vi "play-AFM-CS-imaging_v2.vi"() -> ()   [LabVIEW 2017]
uses:
  z-axis-params.ctl
  controls/boolean_info.ctl
  <userlib>/_matio/level5/Public/MAT-File Data Types.ctl
  <vilib>/userdefined/High Color/nirio_resource_hc.ctl
  controls/expMetaData.ctl
  <vilib>/Utility/file.llb/Read Delimited Spreadsheet (DBL).vi
  <vilib>/FPGAPlugInAG/cRIO-9082/niLvFpga_Open_cRIO-9082.vi
  <vilib>/rvi/interface/common/dynamic/niFpgaDynamicAddResources.vi
  <vilib>/FPGAPlugInAG/Dynamic/niLvFpga_Reset_Dynamic.vi
  <vilib>/rvi/interface/common/niFpgaWaitOnOcc.vi
  <vilib>/Utility/error.llb/Error Cluster From Error Code.vi
  <vilib>/rvi/errors/niLvFpgaAdjustHostInterfaceError.vi
  <vilib>/FPGAPlugInAG/Dynamic/niLvFpga_Run_Dynamic.vi
  <vilib>/Utility/file.llb/Write Delimited Spreadsheet (DBL).vi
  <vilib>/FPGAPlugInAG/Dynamic/niLvFpga_Close_Dynamic.vi
  <userlib>/_matio/level5/Public/Write/Append Data Element.llb/Append Data Element (Anything).vi
  <vilib>/rvi/interface/nirviOpenFPGA/nirviOpenFPGA.xnode
  FPGA Bitfiles/afmimagingcontro_FPGATargetSPARTA_cs-scanningv2.lvbitx
  <vilib>/rvi/interface/nirviMethod/nirviMethod.xnode
  <vilib>/rvi/interface/nirviReadWriteControl/nirviReadWriteControl.xnode
  <vilib>/rvi/interface/nirviCloseFPGA/nirviCloseFPGA.xnode
  <vilib>/FPGAPlugInAG/Dynamic/niLvFpga_ConfigureFifo_Dynamic.vi
  <vilib>/rvi/errors/niLvFpgaMergeErrorWithErrorCode.vi
  <vilib>/rvi/interface/Simulation/niFpgaSimulationCallBeginRW.vi
  <vilib>/FPGAPlugInAG/Dynamic/niLvFpga_ReadFifo_Dynamic.vi
  NiFpgaLv.dll
  <userlib>/_matio/level5.lvlib
  <vilib>/FPGAPlugInAG/Dynamic/niLvFpga_WriteFifo_Dynamic.vi
panel:
  out "xy_ref":fxp<+/-,16,5>[](array[numeric])
  out "xy_k":fxp<+/-,16,5>[](array[numeric])
  out "input-data-path":path
  in  "Kiz_down":sgl=0.001
  in  "max_Z_settle_samples":i16=5000
  out "boolean \nindicators":T1
  out "CS Time":dbl
  out "Current Case":i16
  out "state times":dbl[](array[numeric])
  out "iter":i32
  out "entity-index":i16
  out "x = 0?":bool
  out "Numeric":i32
  out "error out 2":errorcluster
  in  "Tab Control":T2(tab)
  in  "init Z up":sgl step=0.5
  in  "trigger-0":bool
  in  "numEntities":i16
  in  "data-root":path=path "C:/Users/arnold/Documents/labview/afm_imaging/data/cs-data/20microns/parents"
  in  "z-axis-params":T3={"TOL"=0.3, "ramp_rate"=-5e-05, "z_u_max"=5.0, "setpoint"=0.0, "Ki"=0.01, "Z_error_threshold"=0.05, "Z_settled_samples_threshold "=500, "z_UP"=1.5, "zup_N"=500, "TF Order"=1, "Num"=[1.0, 0.0, 0.0, 0.0, 0.0, 0.0, 0.0, 0.0, 0.0], "Den"=[1.0, 0.0, 0.0, 0.0, 0.0, 0.0, 0.0, 0.0, 0.0]} {"Z_error_threshold" format="%#_13g"; "ramp_rate" format="%#_4g"; "TOL" format="%#_13g"}
  in  "step_down_frac":fxp<+,8,1>=1.0
  in  "input-file-name":string="cs-traj-z-bounce.csv"
  out "output-data-path":path
  out "output-meta-data-path":path
  in  "note-blob":string
  in  "overwrite":bool
  in  "TsTicks":u32=1600
  in  "Ki-xy":sgl=0.005
  in  "collect all":bool=TRUE
  in  "collect move":bool
  in  "xy settled-samples\n threshold":i16=200
  in  "xy error-threshold":sgl=0.1
  out "number-settled-samples-x":i16
  out "number-settled-samples-y":i16
  out "case-selected":i16
  out "number-settled-samples-Z":i16
  out "size(s)":i32
  out "nsamps":i32
  out "elements left":i32=1
  out "y iter":i32
  out "size(s) 2":i32[](array[numeric])
  out "Array":i32[][](array[numeric])
  out "z-control":dbl[](graph)
  out "x-axis":dbl[](graph)
  out "z-error":dbl[](graph)
  out "y-axis":dbl[](graph)
  in  "STOP":bool
  # "- If collect all = fasle and collect move = false,\nwe only collect measurement data.\n- If collect all = false, and collect move = true,\nwe collect measurement and move data.\n- If collect all = true, we collect everything."
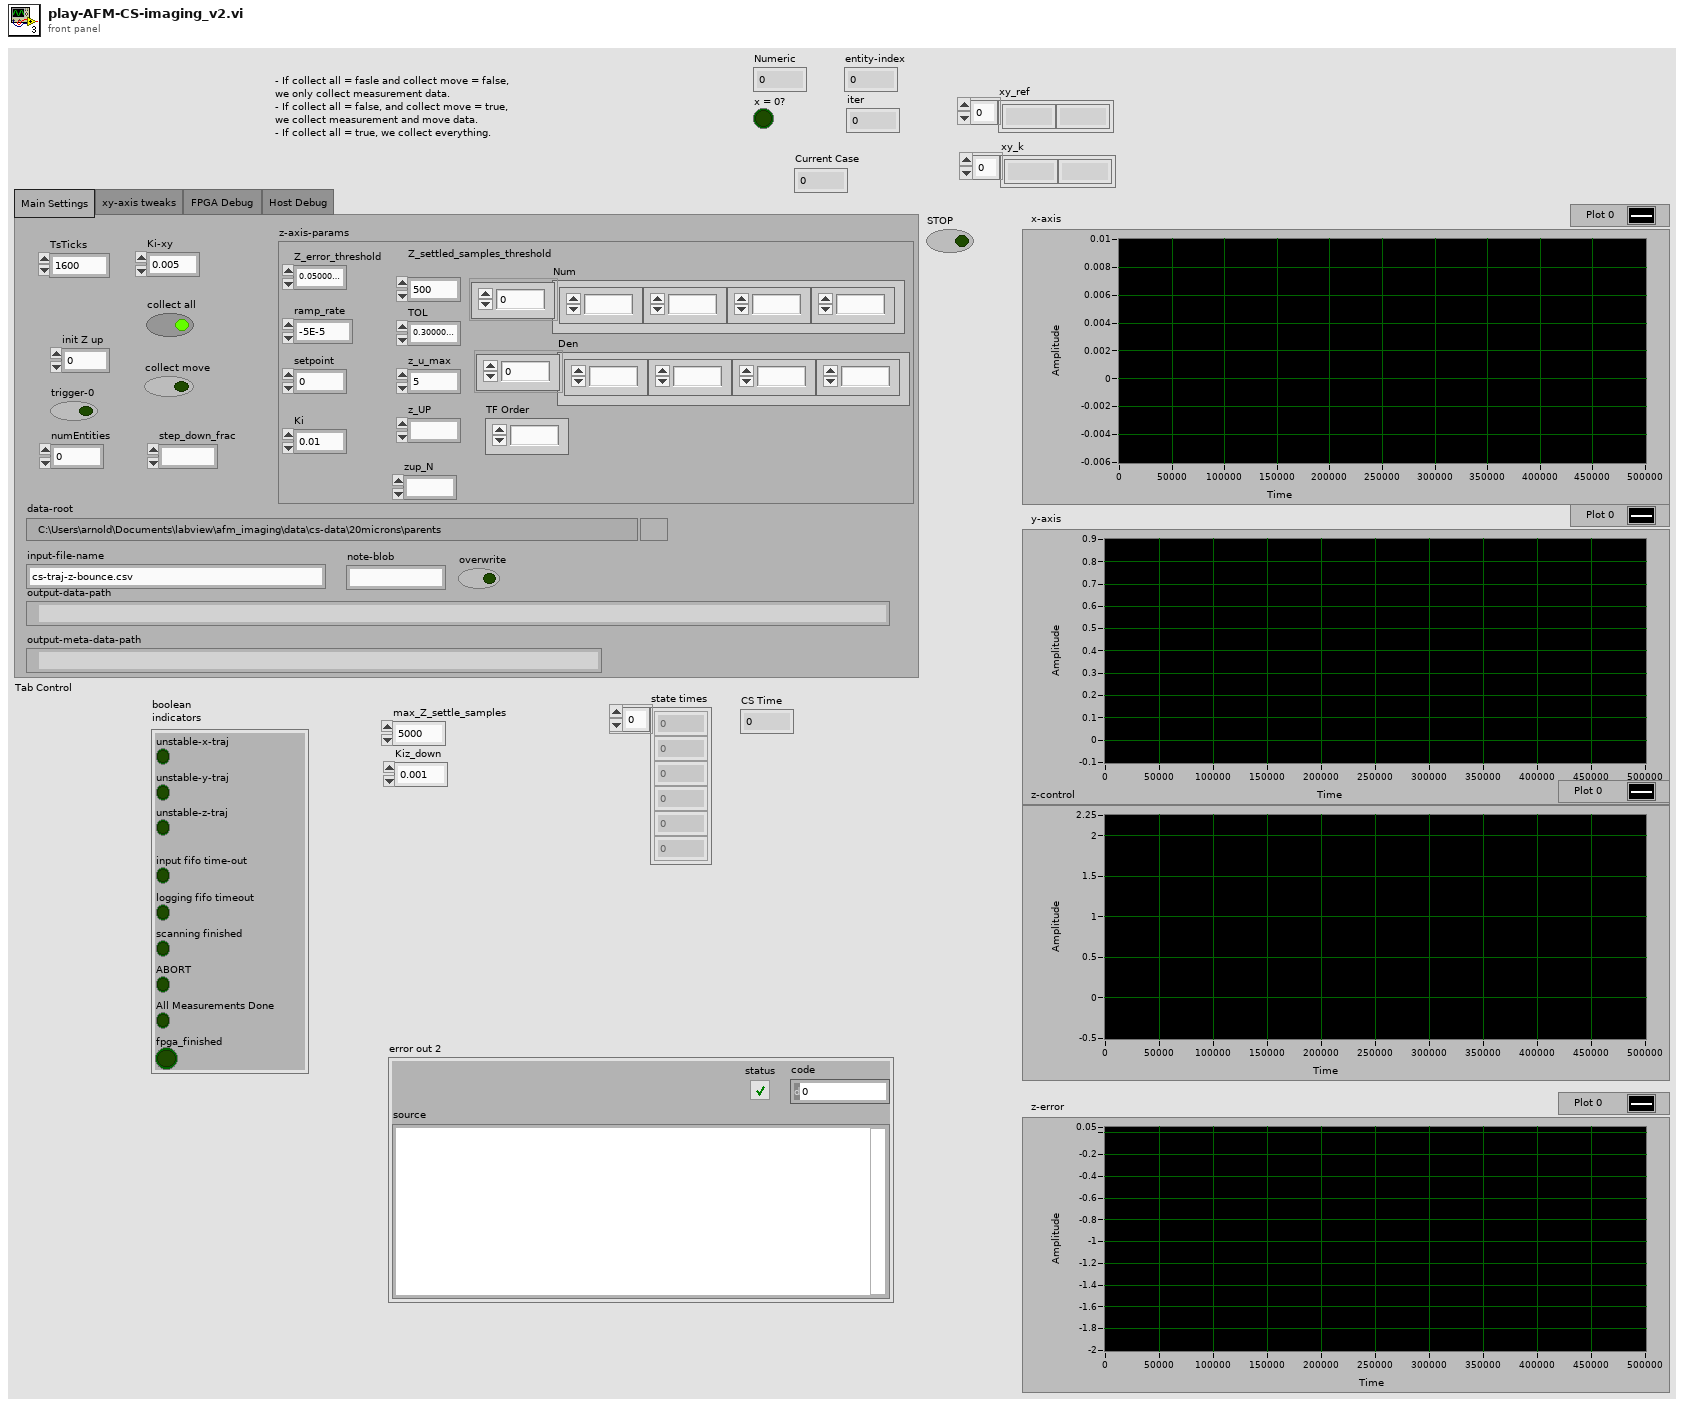
[diagram p1: front panel]
types:
  T1 = typedef "boolean_info.ctl" = cluster{"unstable-z-traj":bool, "input fifo time-out":bool, "logging fifo timeout":bool, "scanning finished":bool, "unstable-x-traj":bool, "unstable-y-traj":bool, "ABORT":bool, "All Measurements Done":bool, "fpga_finished":bool}
  T2 = enum32{"Main Settings", "xy-axis tweaks", "FPGA Debug ", "Host Debug"}
  T3 = typedef "z-axis-params.ctl" = cluster{"TOL":sgl, "ramp_rate":sgl, "z_u_max":sgl, "setpoint":sgl, "Ki":sgl, "Z_error_threshold":sgl, "Z_settled_samples_threshold ":i16, "z_UP":fxp<+/-,16,5>, "zup_N":i16, "TF Order":i32, "Num":sgl[], "Den":sgl[]}
  T4 = typedef "level5.lvlib/MAT-File Data Types.ctl" = enum32{"_invalid", "miINT8", "miUINT8", "miINT16", "miUINT16", "miINT32", "miUINT32", "miSINGLE", "_reserved_1", "miDOUBLE", "_reserved_2", "_reserved_3", "miINT64", "miUINT64", "miMATRIX", "miCOMPRESSED", "miUTF8", "miUTF16", "miUTF32"}
  T5 = typedef "nirio_resource_hc.ctl" = tag
  T6 = cluster{"unstable-z-traj":bool, "input fifo time-out":bool, "logging fifo timeout":bool, "scanning finished":bool, "unstable-x-traj":bool, "unstable-y-traj":bool, "ABORT":bool, "All Measurements Done":bool, "fpga_finished":bool}
  T7 = enum16{"open", "replace", "create", "open or create", "replace or create", "replace or create with confirmation"}
  T8 = typedef "expMetaData.ctl" = cluster{"xy_error_threshold":sgl, "xy_settled_samples_threshold":i16, "Ki_xy":sgl, "state_counts":dbl[], "TOL":sgl, "ramp_rate":sgl, "z_u_max":sgl, "setpoint":sgl, "Ki":sgl, "Z_error_threshold":sgl, "Z_settled_samples_threshold ":i16, "z_UP":sgl, "zup_N":i16, "Num":sgl[], "Den":sgl[], "max_Z_settle_samples":i16, "Kiz_down":sgl, "do_xy_CL":bool, "do_Alt_Ztrigger":bool, "output-data-path":path, "input-data-path":path}
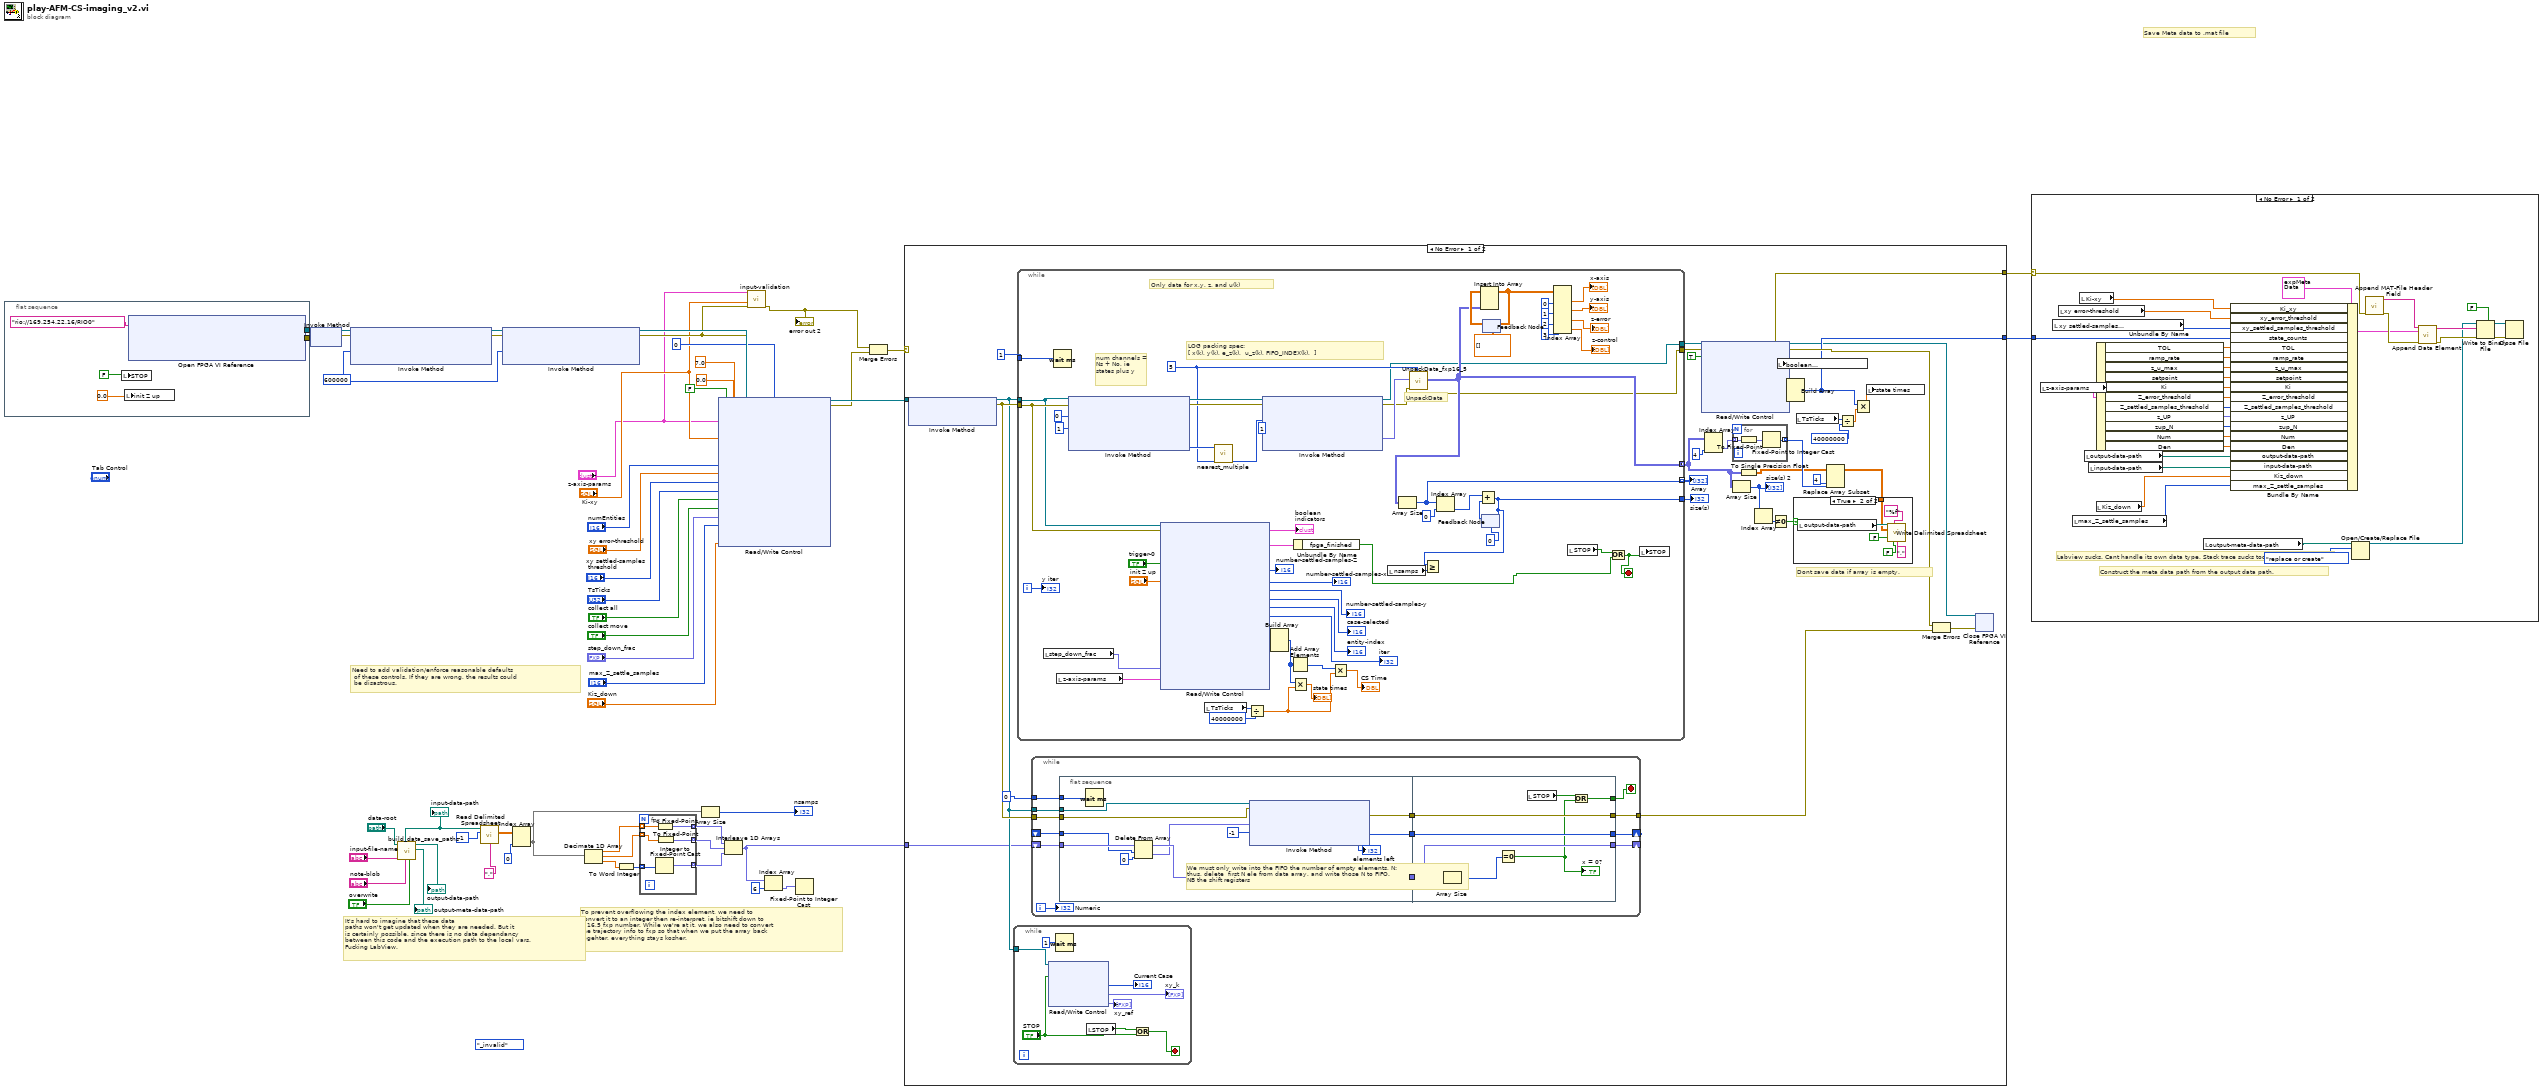
[diagram p0: block diagram]
diagram:
  (unwired) MAT-File_Data_Types."_invalid" ("MAT-File Data Types")
  w52 = 600000
  # "It's hard to imagine that these data\npaths won't get updated when they are needed. But it \nis certainly possible, since there is no data dependancy \nbetween this code and the execution path to the local vars.\nFucking LabView."
  # "Save Meta data to .mat file"
  # "To prevent overflowing the index element, we need to \nconvert it to an integer then re-interpret, ie bitshift down to \na 16,5 fxp number. While we're at it, we also need to convert\nthe trajectory info to fxp so that when we put the array back\ntogehter, everything stays kosher."
  # "Need to add validation/enforce reasonable defaults\n of these controls. If they are wrong, the results could\n be disastrous."
  n1 = flat-sequence {
    tunnel: [w58] -> w51
    tunnel: [w57] -> w50
    frame #0 {
      n2 = local write "STOP"(FALSE) -> ()
      n3 = local write "init Z up"(0.0) -> ()
      n4 = xnode "Open FPGA VI Reference"("resource name"=T5 "rio://169.254.22.16/RIO0") -> ("FPGA VI Reference Out"=w58:refnum<k20>, "error out"=w57:errorcluster)  [unwired: 1 in]
    }
  }
  n5 = xnode "Invoke Method"("FPGA VI Reference In"=w51, "error in"=w50) -> ("FPGA VI Reference Out"=w45:refnum<k20>, "error out"=w44:errorcluster)
  n6 = xnode "Invoke Method"("FPGA VI Reference In"=w45, "error in"=w44, "Requested Depth"=w52) -> ("FPGA VI Reference Out"=w47:refnum<k20>, "error out"=w48:errorcluster)  [unwired: 1 out]
  n7 = call "build_data_save_paths.vi"("overwrite"="overwrite", "note-blob"="note-blob", "base-file-name"="input-file-name", "data-root"="data-root") -> ("output-meta-data-path"=→"output-meta-data-path":path, "output-data-path"=→"output-data-path":path, "input-data-path"=w6:path)  [unwired: 3 in, 2 out]
  "input-data-path" <- w6
  n8 = call-poly <vilib>:"Read Delimited Spreadsheet.vi"("file path (dialog if empty)"=w6, "number of rows (all:-1)"=-1, "delimiter (\\t)"=",") -> ("all rows"=w39:dbl[][])  [unwired: 7 in, 5 out]
  n9 = xnode "Invoke Method"("FPGA VI Reference In"=w47, "error in"=w48, "Requested Depth"=w52) -> ("FPGA VI Reference Out"=w53:refnum<k20>, "error out"=w31:errorcluster)  [unwired: 1 out]
  n10 = Index Array(array=w39, index (col)=0 ("dimension size")) -> (element=w17:dbl[])  [unwired: 1 in]
  n11 = Decimate 1D Array(w17) -> (w25:dbl[], w24:dbl[], w26:dbl[])
  n12 = To Word Integer(number=w26) -> (16bit integer=w23:i16[])
  n13 = for {
    tunnel: w25 -> [w64] mode=indexing
    tunnel: w24 -> [w63] mode=indexing
    tunnel: [w62] -> w21 mode=indexing
    tunnel: [w61] -> w22 mode=indexing
    tunnel: w23 -> [w60] mode=indexing
    tunnel: [w59] -> w20 mode=indexing
    n14 = Integer to Fixed-Point Cast(integer=w60) -> (fixed-point=w59:fxp<+/-,16,5>)  [unwired: 1 in]
    n15 = To Fixed-Point(number=w64) -> (fixed-point=w61:fxp<+/-,16,5>)  [unwired: 1 in]
    n16 = To Fixed-Point(number=w63) -> (fixed-point=w62:fxp<+/-,16,5>)  [unwired: 1 in]
  }
  n17 = Array Size(array=w17) -> (size(s)=→"nsamps":i32)
  n18 = xnode "Read/Write Control"("FPGA VI Reference In"=w53, "error in"=w31, "initial case"=i16 0, "z-axis-params"="z-axis-params", "xy-bound"=sgl 7.0, "Ki-xy"="Ki-xy", "init Z up"=sgl 0.0 ("u(0)"), "trigger-0"=FALSE, "numEntities"="numEntities", "xy-error-threshold"="xy error-threshold", "settled-samples threshold"="xy settled-samples\n threshold", "TsTicks"="TsTicks", "collect all"="collect all", "collect move"="collect move", "step_down_frac"="step_down_frac", "max_Z_settle_samples"="max_Z_settle_samples", "Kiz_down"="Kiz_down") -> ("FPGA VI Reference Out"=w46:refnum<k20>, "error out"=w28:errorcluster)  [unwired: 1 out]
  n19 = Interleave 1D Arrays(w22, w21, w20) -> (w16:fxp<+/-,16,5>[])
  n20 = call "input-validation.vi"("error constant"=w31, "Ki-xy"="Ki-xy", "z-axis-params"="z-axis-params") -> ("error out"=w27:errorcluster)  [unwired: 8 in]
  "error out 2" <- w27
  n21 = Index Array(array=w16, index=6) -> (element=w19:fxp<+/-,16,5>)
  n22 = Fixed-Point to Integer Cast(1:w19) -> ()  [unwired: 1 out]
  n23 = Merge Errors(w27, w28) -> (w1:errorcluster)
  n24 = case shown="No Error" w1 {
    selector: w1 -> [_ w209]
    tunnel: w46 -> [w99 _]
    tunnel: w16 -> [w97 _]
    tunnel: [w96 w209] -> w13
    tunnel: [w95 _] -> w12
    frame No Error {
      # "Dont save data if array is empty."
      n25 = xnode "Invoke Method"("FPGA VI Reference In"=w99) -> ("FPGA VI Reference Out"=w98:refnum<k20>, "error out"=w100:errorcluster)  [unwired: 2 in]
      n26 = while {
        tunnel: w98 -> [w117]
        stop <- w113 stop-if-true
        n27 = xnode "Read/Write Control"("FPGA VI Reference In"=w117, "ABORT"="STOP") -> ("Current Case"=→"Current Case":u8, "xy_k"=→"xy_k":fxp<+/-,16,5>[], "xy_ref"=→"xy_ref":fxp<+/-,16,5>[])  [unwired: 1 in, 2 out]
        n28 = Wait (ms)(milliseconds to wait=u32 1) -> ()  [unwired: 1 out]
        n29 = local read "STOP"() -> (w114:bool)
        n30 = Or(x=w114, y="STOP") -> (x .or. y?=w113:bool)
      }
      n31 = while {
        tunnel: 1 -> [w208]
        tunnel: w98 -> [w196]
        tunnel: w100 -> [w197]
        tunnel: [w161] -> w89
        tunnel: [w172] -> w80 mode=concatenating
        tunnel: [w194] -> w93
        tunnel: [w170] -> w88
        tunnel: [w187] -> w85 mode=indexing
        i -> [w195]
        stop <- w188 stop-if-true
        w173 = u32 5 ("y")
        # "LOG packing spec:\n[ x(k), y(k), e_z(k),  u_z(k), FIFO_INDEX(k),  ]"
        # "num channels = Ns + No, ie states plus y"
        # "Only data for x,y, z, and u(k)"
        # "UnpackData"
        n32 = local read "step_down_frac"() -> (w149:fxp<+,8,1>)
        n33 = Wait (ms)(milliseconds to wait=w208) -> ()  [unwired: 1 out]
        n34 = local read "z-axis-params"() -> (w150:T3)
        n35 = xnode "Invoke Method"("FPGA VI Reference In"=w196, "error in"=w197, "Number of Elements"=0 ("Timeout (ms)"), "Timeout (ms)"=1) -> ("FPGA VI Reference Out"=w204:refnum<k20>, "error out"=w205:errorcluster, "Elements Remaining"=w191:u32)  [unwired: 1 out]
        n36 = xnode "Read/Write Control"("FPGA VI Reference In"=w196, "error in"=w197, "trigger-0"="trigger-0", "init Z up"="init Z up", "step_down_frac"=w149, "z-axis-params"=w150) -> ("boolean  indicators"=w154:T6, "number-settled-samples-Z"=→"number-settled-samples-Z":i16, "number-settled-samples-x"=→"number-settled-samples-x":i16, "number-settled-samples-y"=→"number-settled-samples-y":i16, "Current Case"=→"case-selected":u8, "entity-index"=→"entity-index":i16, "iter"=→"iter":i32, "state1-count"=w166:u64, "state2-count"=w165:u64, "state3-count"=w164:u64, "state4-count"=w163:u64, "state5-count"=w162:u64)  [unwired: 1 in, 3 out]
        "boolean \nindicators" <- w154
        n37 = local read "TsTicks"() -> (w157:u32)
        n38 = call "nearest_multiple.vi"("numChan"=w173, "N"=w191) -> ("(int) y*floor(x/y)"=w190:u64)  [unwired: 9 in]
        n39 = Divide(x=w157, y=u32 40000000) -> (x/y=w152:dbl)
        n40 = xnode "Invoke Method"("FPGA VI Reference In"=w204, "error in"=w205, "Number of Elements"=w190, "Timeout (ms)"=1) -> ("FPGA VI Reference Out"=w161:refnum<k20>, "error out"=w170:errorcluster, "Data"=w171:fxp<+/-,16,5>[])  [unwired: 1 out]
        n41 = Build Array(w166, w165, w164, w163, w162) -> (w153:u64[])
        n42 = Add Array Elements(numeric array=w153) -> (sum=w158:u64)
        n43 = Multiply(x=w153, y=w152) -> (x*y=→"state times":dbl[])
        n44 = Unbundle By Name(w154) -> ("fpga_finished"=w169:bool)
        n45 = Multiply(x=w158, y=w152) -> (x*y=→"CS Time":dbl)
        n46 = local read "nsamps"() -> (w201:i32)
        n47 = call "UnpackData_fxp16_5.vi"("NumChannels"=w173, "error In"=w170, "1D Data In"=w171) -> ("2D Data Out"=w172:fxp<+/-,16,5>[][])  [unwired: 7 in, 1 out]
        n48 = Array Size(array=w172) -> (size(s)=w187:i32[])
        n49 = Index Array(array=w187, index=0) -> (element=w199:i32)
        n50 = feedback #1(0) -> (w200:i32)
        n51 = Add(x=w199, y=w200) -> (x+y=w194:i32)
        n52 = Greater Or Equal?(x=w194, y=w201) -> ()  [unwired: 1 out]
        n53 = feedback-in #1(w194) -> ()
        n54 = feedback #2(dbl[][] []) -> (w183:dbl[][])
        n55 = Insert Into Array(array=w183, new element=w172) -> (w174:dbl[][])  [unwired: 2 in]
        n56 = feedback-in #2(w174) -> ()
        n57 = Index Array(array=w174, index (col) #1=0 ("disabled index (col)"), index (col) #2=1 ("index (col)"), index (col) #3=2 ("index (col)"), index (col) #4=3 ("index (col)")) -> (element #1=→"x-axis":dbl[], element #2=→"y-axis":dbl[], element #3=→"z-error":dbl[], element #4=→"z-control":dbl[])  [unwired: 4 in]
        n58 = local read "STOP"() -> (w189:bool)
        n59 = Or(x=w189, y=w169) -> (x .or. y?=w188:bool)
        n60 = local write "STOP"(w188) -> ()
        "y iter" <- w195
      }
      "size(s)" <- w93
      "Array" <- w85
      n61 = while {
        tunnel: [w128] -> w90
        tunnel: 0 -> [w130]
        shift-right: [w124] -> _
        shift-left: _ -> [w127]
        shift-right: [w122] -> _
        shift-left: w97 -> [w129]
        tunnel: w98 -> [w121]
        tunnel: w100 -> [w120]
        i -> [w118]
        stop <- w119 stop-if-true
        n62 = flat-sequence {
          tunnel: w130 -> [w141]
          tunnel: w129 -> [w136]
          tunnel: w127 -> [w132]
          tunnel: [w139] -> w126
          tunnel: [w137] -> w125
          tunnel: [w138] -> w123
          tunnel: w121 -> [w134]
          tunnel: w120 -> [w133]
          tunnel: [w148] -> w124
          tunnel: [w145] -> w128
          tunnel: w126 -> [w145]
          tunnel: w125 -> [w148]
          tunnel: w123 -> [w146]
          tunnel: [w146] -> w122
          tunnel: [w142] -> w119
          frame #0 {
            # "We must only write into the FIFO the number of empty elements, N:\nthus, delete  first N ele from data array, and write those N to FIFO.\nNB the shift registers"
            n63 = Wait (ms)(milliseconds to wait=w141) -> ()  [unwired: 1 out]
            n64 = Delete From Array(array=w136, length=w132, index=0) -> (deleted portion=w135:fxp<+/-,16,5>[], array with subset deleted=w138:fxp<+/-,16,5>[])
            n65 = xnode "Invoke Method"("FPGA VI Reference In"=w134, "error in"=w133, "Data"=w135, "Timeout (ms)"=-1) -> ("error out"=w139:errorcluster, "Empty Elements Remaining"=w137:u32)  [unwired: 1 out]
            "elements left" <- w137
          }
          frame #1 {
            n66 = Array Size(array=w146) -> (size(s)=w147:i32)
            n67 = Equal To 0?(x=w147) -> (x = 0?=w144:bool)
            "x = 0?" <- w144
            n68 = local read "STOP"() -> (w143:bool)
            n69 = Or(x=w143, y=w144) -> (x .or. y?=w142:bool)
          }
        }
        "Numeric" <- w118
      }
      n70 = xnode "Read/Write Control"("FPGA VI Reference In"=w89, "error in"=w88, "ABORT"=TRUE) -> ("FPGA VI Reference Out"=w86:refnum<k20>, "error out"=w96:errorcluster, "boolean  indicators"=w69:T6, "state1-count"=w78:u64, "state2-count"=w77:u64, "state3-count"=w76:u64, "state4-count"=w75:u64, "state5-count"=w74:u64)
      n71 = Index Array(array=w80, index (col)=4) -> (element=w83:fxp<+/-,16,5>[])  [unwired: 1 in]
      n72 = for {
        tunnel: w83 -> [w108] mode=indexing
        tunnel: [w109] -> w81 mode=indexing
        n73 = To Fixed-Point(number=w108) -> (fixed-point=w107:fxp<+/-,16,5>)  [unwired: 1 in]
        n74 = Fixed-Point to Integer Cast(1:w107) -> (0:w109:i16)
      }
      n75 = Array Size(array=w80) -> (size(s)=w70:i32[])
      "size(s) 2" <- w70
      n76 = To Single Precision Float(number=w80) -> (single precision float=w79:sgl[][])
      n77 = Index Array(array=w70) -> (element=w71:i32)  [unwired: 1 in]
      n78 = Not Equal To 0?(x=w71) -> (x != 0?=w72:bool)
      n79 = local write "boolean \nindicators"(w69) -> ()
      n80 = Build Array(w78, w77, w76, w75, w74) -> (w95:u64[])
      n81 = local read "TsTicks"() -> (w68:u32)
      n82 = Replace Array Subset(array=w79, new element=w81, index (col)=4) -> (w73:sgl[][])  [unwired: 1 in]
      n83 = case shown="True" w72 {
        tunnel: w73 -> [_ w101]
        frame False {
        }
        frame True {
          n84 = local read "output-data-path"() -> (w106:path)
          n85 = call-poly <vilib>:"Write Delimited Spreadsheet.vi"("file path (dialog if empty)"=w106, "format (%.3f)"="%f", "2D data"=w101, "append to file? (new file:F)"=FALSE, "transpose? (no:F)"=FALSE, "delimiter (\\t)"=",") -> ()  [unwired: 8 in, 2 out]
        }
      }
      n86 = Divide(x=w68, y=u32 40000000) -> (x/y=w66:dbl)
      n87 = Multiply(x=w95, y=w66) -> (x*y=w65:dbl[])
      n88 = local write "state times"(w65) -> ()
      n89 = Merge Errors(w96, w90) -> (w91:errorcluster)
      n90 = xnode "Close FPGA VI Reference"("FPGA VI Reference In"=w86, "error in"=w91) -> ()  [unwired: 1 out]
    }
    frame Error {
    }
  }
  n91 = case shown="No Error" w13 {
    selector: w13 -> [w235 _]
    tunnel: w12 -> [w222 _]
    frame No Error {
      # "Construct the meta data path from the output data path."
      # "Labview sucks. Cant handle its own data type. Stack trace sucks too."
      n92 = local read "z-axis-params"() -> (w221:T3)
      n93 = local read "xy settled-samples\n threshold"() -> (w218:i16)
      n94 = local read "xy error-threshold"() -> (w219:sgl)
      n95 = local read "max_Z_settle_samples"() -> (w211:i16)
      n96 = local read "Ki-xy"() -> (w220:sgl)
      n97 = local read "output-data-path"() -> (w213:path)
      n98 = local read "input-data-path"() -> (w212:path)
      n99 = Unbundle By Name(w221) -> ("TOL"=w232:sgl, "ramp_rate"=w231:sgl, "z_u_max"=w230:sgl, "setpoint"=w229:sgl, "Ki"=w228:sgl, "Z_error_threshold"=w227:sgl, "Z_settled_samples_threshold"=w226:i16, "z_UP"=w225:fxp<+/-,16,5>, "zup_N"=w224:i16, "Num"=w215:sgl[], "Den"=w214:sgl[])
      n100 = local read "Kiz_down"() -> (w210:sgl)
      n101 = local read "output-meta-data-path"() -> (w216:path)
      n102 = Bundle By Name(cluster=T8 {"xy_error_threshold"=0.1, "xy_settled_samples_threshold"=200, "Ki_xy"=0.005, "state_counts"=[], "TOL"=0.3, "ramp_rate"=-5e-06, "z_u_max"=5.0, "setpoint"=0.0, "Ki"=0.001, "Z_error_threshold"=0.0, "Z_settled_samples_threshold "=0, "z_UP"=1.5, "zup_N"=5000, "Num"=[-0.00254, 0.000408, 0.00295, 0.0, 0.0, 0.0, 0.0, 0.0, 0.0], "Den"=[0.982758, -1.98194, 1.0, 0.0, 0.0, 0.0, 0.0, 0.0, 0.0], "max_Z_settle_samples"=5000, "Kiz_down"=0.001, "do_xy_CL"=FALSE, "do_Alt_Ztrigger"=FALSE, "output-data-path"=path "", "input-data-path"=path ""} ("ExpMetaData"), "Ki_xy"=w220, "xy_error_threshold"=w219, "xy_settled_samples_threshold"=w218, "state_counts"=w222, "TOL"=w232, "ramp_rate"=w231, "z_u_max"=w230, "setpoint"=w229, "Ki"=w228, "Z_error_threshold"=w227, "Z_settled_samples_threshold"=w226, "z_UP"=w225, "zup_N"=w224, "Num"=w215, "Den"=w214, "output-data-path"=w213, "input-data-path"=w212, "Kiz_down"=w210, "max_Z_settle_samples"=w211) -> (w233:T8)
      n103 = Open/Create/Replace File(file path (use dialog)=w216, operation (0:open)=T7."replace or create") -> (refnum out=w234:refnum<file>)  [unwired: 4 in, 2 out]
      n104 = call <userlib>:"Append MAT-File Header Field.vi"("error"=w235) -> ("result string"=w242:string, "error out"=w236:errorcluster)  [unwired: 13 in]
      n105 = call-poly <userlib>:"Append Data Element.vi"("initial string"=w242, "data"=w233, "error in (no error)"=w236) -> ("result string"=w240:string, "error out"=w241:errorcluster)  [unwired: 11 in]
      n106 = Write to Binary File(file (use dialog)=w234, data=w240, error in=w241, 5:FALSE ("prepend array or string size? (T)")) -> (refnum out=w237:refnum<file>, error out=w238:errorcluster)  [unwired: 2 in, 1 out]
      n107 = Close File(refnum=w237, error in=w238) -> ()  [unwired: 2 out]
    }
    frame Error {
    }
  }
